vi "check parameters.vi"(8 "error in (no error)":errorcluster, 11 "Request in":variant) -> (0 "error out":errorcluster, 3 "Request out":variant)   [LabVIEW 2017, in "JSONRPC Server.lvclass"]
uses:
  JSONRPC Server.lvclass
  <vilib>/National Instruments/Variant Data Manipulation/Variant Data Manipulation.lvlib
  <vilib>/Utility/Data Type/NI_Data Type.lvlib
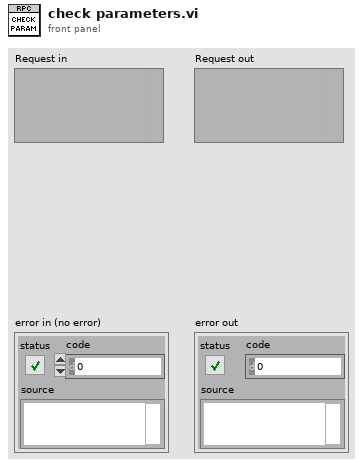
[diagram p1: front panel]
types:
  T1 = typedef "NI_Data Type.lvlib/Data Type.ctl" = enum8{"Invalid Type", "Void", "I8", "I16", "I32", "I64", "U8", "U16", "U32", "U64", "Single Float", "Double Float", "Extended Float", "Single Complex", "Double Complex", "Extended Complex", "Enum U8", "Enum U16", "Enum U32", "Enum U64", "Single Float With Unit", "Double Float With Unit", "Extended Float With Unit", "Single Complex with Unit", "Double Complex with Unit", "Extended Complex with Unit", "Boolean", "String", "Path", "Picture", "Tag", "Array", "Cluster", "Variant", "LV Variant", "Waveform", "Timestamp", "Digital Waveform", "Digital Data", "ExpressData", "Refnum", "External Data", "VI", "Poly VI", "LabVIEW Class Instance", "Fixed Point"}
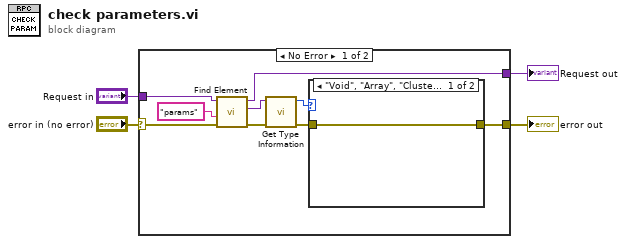
[diagram p0: block diagram]
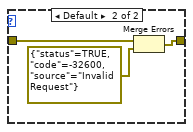
[diagram p2: hidden frame]
diagram:
  n1 = case shown="No Error" "error in (no error)" {
    selector: "error in (no error)" -> [w11 w18]
    tunnel: "Request in" -> [w13 w19]
    tunnel: [w9 w19] -> w2
    tunnel: [w7 w18] -> w1
    frame No Error {
      n2 = call <vilib>:"Find Element.vi"("error in (no error)"=w11, "Name"="params", "Variant (Cluster) in"=w13) -> ("error out"=w12:errorcluster, "element"=w8:variant, "Variant (Cluster) out"=w9:variant)  [unwired: 4 in, 2 out]
      n3 = call <vilib>:"Get Type Information.vi"("error in (no error)"=w12, "Variant"=w8) -> ("error out"=w5:errorcluster, "Type"=w6:T1)  [unwired: 5 in, 3 out]
      n4 = case shown="\"Void\", \"Array\", \"Cluster\"" w6 {
        tunnel: [w14 w16] -> w7
        tunnel: w5 -> [w14 w15]
        frame "Void", "Array", "Cluster" {
        }
        frame Default {
          n5 = Merge Errors(w15, errorcluster {"status"=TRUE, "code"=-32600, "source"="Invalid Request"} ("error IO")) -> (w16:errorcluster)
        }
      }
    }
    frame Error {
    }
  }
  "error out" <- w1
  "Request out" <- w2
